vi "Module ID.vi"(11 "GUIHandler in":refnum<class "GUIHandler.lvclass">) -> (2 "Module ID":string)   [LabVIEW 2020, in "VolatusGUI.lvlib" / "GUIHandler.lvclass"]
uses:
  GUIHandler.lvclass
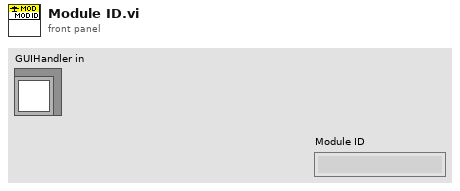
[diagram p1: front panel]
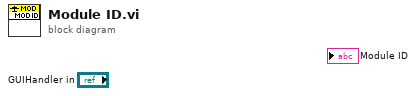
[diagram p0: block diagram]
diagram:
